vi "H5Pget_version.vi"(8 "error in (no error)":errorcluster, 11 "HDF5 Property List Ref":T1) -> (0 "error out":errorcluster, 1 "Symbol Table":u32, 2 "Freelist":u32, 3 "HDF5 Property List Ref out":T1, 4 "Shared Object Header":u32, 5 "Super Block":u32)   [LabVIEW 2017]
doc: "Retrieves the version information of various objects for \n a file creation property list."
uses:
  <vilib>/UPVI/lvhdf5/library.llb/HDF5 Ref.ctl
  <vilib>/UPVI/lvhdf5/hdf5.dll
panel:
  # "LVHDF5 Toolkit\nCopyright (c) 2005-2013 by Jason D. Sommerville\nCopyright (c) 2014 by UPVI, LLC.\n\nThis use and distribution of this file is governed by the terms found in \nLICENSE.txt distributed with this toolkit and installed at\n <user.lib>\\_lvhdf5\\LICENSE.txt"
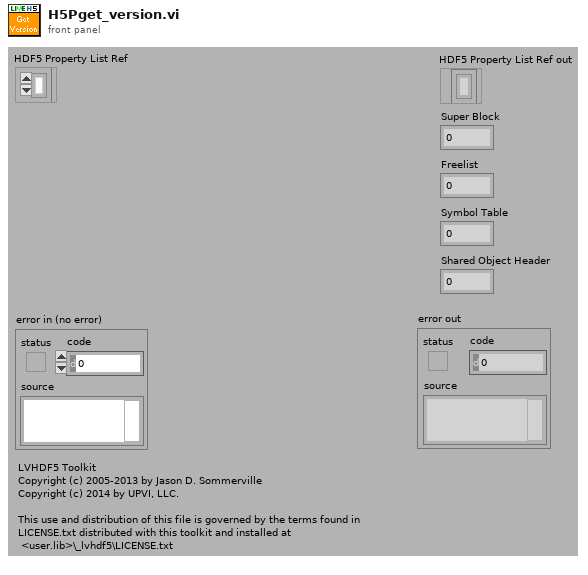
[diagram p1: front panel]
types:
  T1 = typedef "HDF5 Ref.ctl" = refnum<k1>
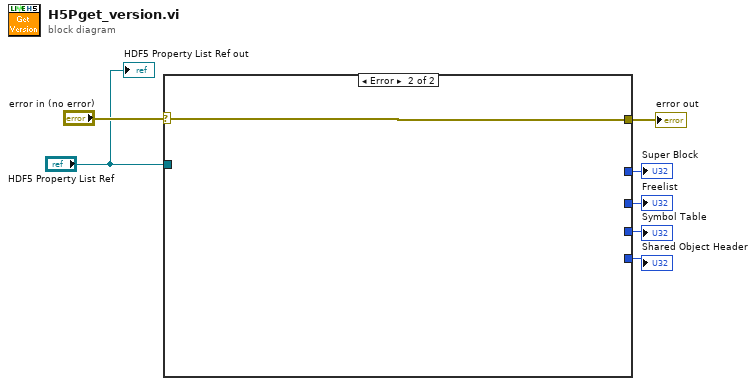
[diagram p0: block diagram]
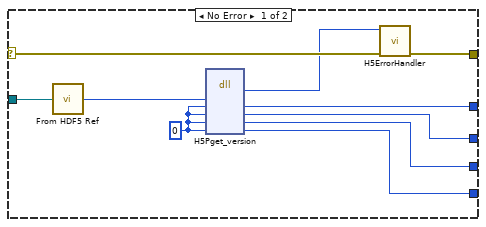
[diagram p2: hidden frame]
diagram:
  n1 = case shown="Error" "error in (no error)" {
    selector: "error in (no error)" -> [w17 w18]
    tunnel: [w16 w18] -> w6
    tunnel: "HDF5 Property List Ref" -> [w15 _]
    tunnel: [w11 _] -> w4
    tunnel: [w10 _] -> w3
    tunnel: [w9 _] -> w2
    tunnel: [w8 _] -> w1
    frame No Error {
      w12 = u32 0
      n2 = call <vilib>:"From HDF5 Ref.vi"("HDF5 Ref"=w15) -> ("I32"=w14:i32)
      n3 = dll-call lib="C:/Program Files/National Instruments/LabVIEW 2017/vi.lib/UPVI/lvhdf5/hdf5.dll" fn="H5Pget_version"("plist_id"=w14, "super"=w12, "freelist"=w12, "stab"=w12, "shhdr"=w12) -> (w13:i32, "super"=w11:u32, "freelist"=w10:u32, "stab"=w9:u32, "shhdr"=w8:u32)  [unwired: 4 in, 2 out]
      n4 = call <vilib>:"H5ErrorHandler.vi"("error in (no error)"=w17, "herr_t"=w13) -> ("error out"=w16:errorcluster)  [unwired: 3 in, 4 out]
    }
    frame Error {
    }
  }
  "error out" <- w6
  "Super Block" <- w4
  "Freelist" <- w3
  "Symbol Table" <- w2
  "Shared Object Header" <- w1
  "HDF5 Property List Ref out" <- "HDF5 Property List Ref"
